vi "lj_stop.vi"(8 "error in":errorcluster, 11 "Handle":i32) -> (0 "error out":errorcluster, 3 "Handle Out":i32)   [LabVIEW 2025, in "LabJackEKG.lvlib"]
uses:
  LabJackEKG.lvlib
panel:
  # "LabJack V0.10\nClose"
  # "09.05.2025"
  # "Blaz Kelbl"
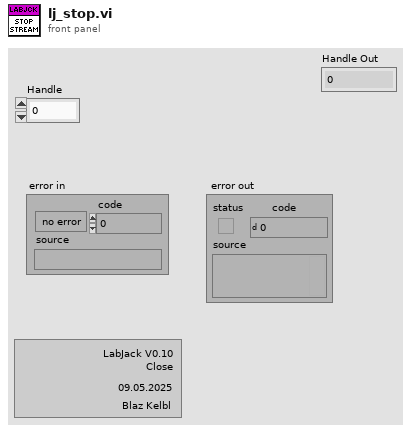
[diagram p1: front panel]
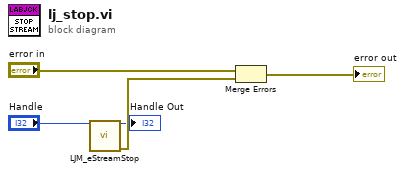
[diagram p0: block diagram]
diagram:
  n1 = call <vilib>:"LJM_eStreamStop.vi"("Handle In"="Handle") -> ("Handle Out"=→"Handle Out":i32, "error out"=w5:errorcluster)  [unwired: 13 in]
  n2 = Merge Errors("error in", w5) -> (→"error out":errorcluster)
